vi "Stop All Plugins.vi"(8 "error in (no error)":errorcluster, 11 "CIFPluginLoader in":refnum<class "CIFPluginLoader.lvclass">) -> (0 "error out":errorcluster, 3 "CIFPluginLoader out":refnum<class "CIFPluginLoader.lvclass">)   [LabVIEW 2021, in "CIFPluginLoader.lvclass"]
uses:
  CIFPluginLoader.lvclass
  CIFPluginLoader.lvclass/CIFPluginLoader.ctl
  CIFUtilities/CIFLogs/Typedef/Message Type.ctl
  typedef/Loaded Plugin Map.ctl
  <vilib>/gRPC/LabVIEW gRPC Library/Client API/Close Client.vi
  CIFCore/Grpc/CIFCoreWrapper/CIFCoreWrapper.lvlib
  CIFUtilities/CIFLogs/CIFLogs.lvlib
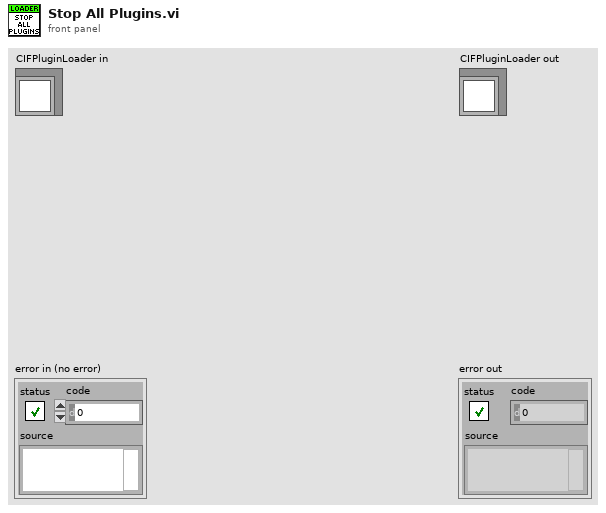
[diagram p1: front panel]
types:
  T1 = typedef "CIFPluginLoader.lvclass/Loaded Plugin Map.ctl" = map{string, refnum<vi>}
  T2 = typedef "grpc-lvsupport-release.lvlib/grpcId.ctl" = u64
  T3 = typedef "CIFLogs.lvlib/Message Type.ctl" = enum16{"Error", "Information", "Print Terminal", "Configuration"}
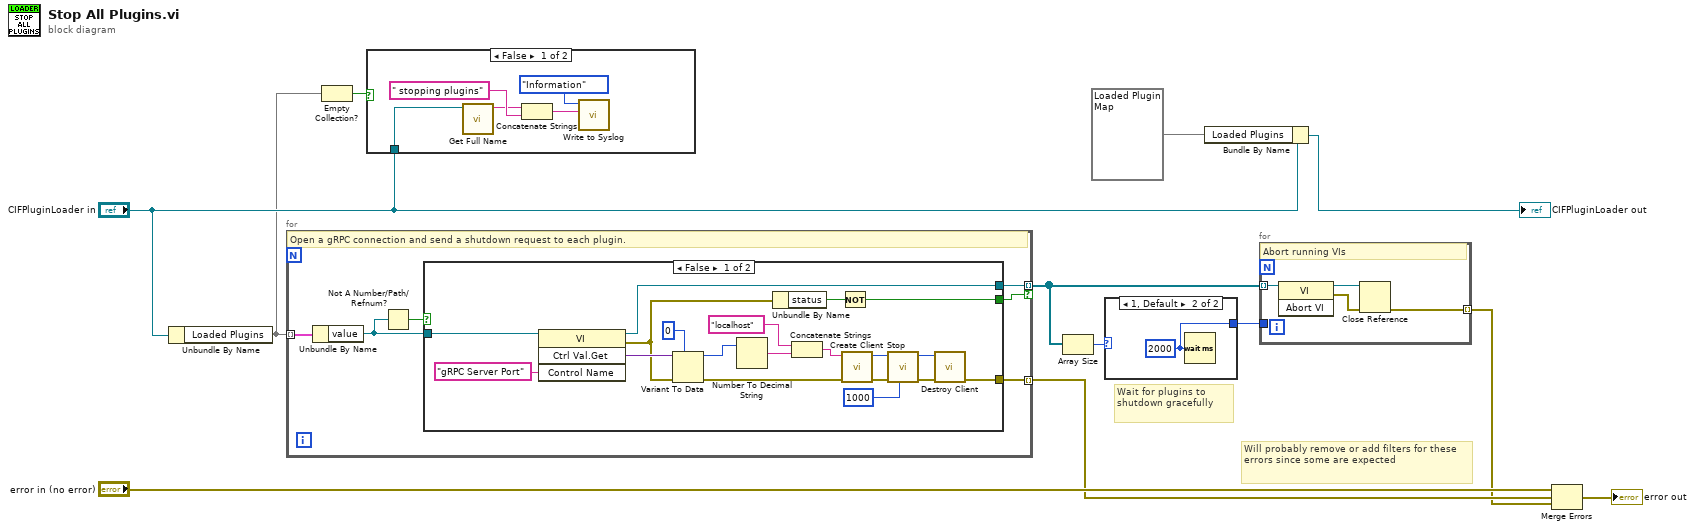
[diagram p0: block diagram]
diagram:
  # "Wait for plugins to shutdown gracefully"
  # "Will probably remove or add filters for these errors since some are expected"
  n1 = Unbundle By Name("CIFPluginLoader in") -> ("Loaded Plugins"=w1:T1)
  n2 = for {
    tunnel: w1 -> [w17] mode=indexing
    tunnel: [w15] -> w12 mode=indexing if=w14
    tunnel: [w13] -> w8 mode=indexing
    # "Open a gRPC connection and send a shutdown request to each plugin."
    n3 = Unbundle By Name(w17) -> ("value"=w16:refnum<vi>)
    n4 = Not A Number/Path/Refnum?(number/path/refnum=w16) -> (NaN/Path/Refnum?=w18:bool)
    n5 = case shown="False" w18 {
      tunnel: w16 -> [w36 _]
      tunnel: [w23 _] -> w15
      tunnel: [w20 _] -> w14
      tunnel: [w19 _] -> w13
      frame False {
        n6 = invoke class="VI" method="Ctrl Val.Get"(reference=w36, "Control Name"="gRPC Server Port") -> (reference out=w23:refnum<vi>, error out=w22:errorcluster, "Get Control Value Variant"=w35:variant)  [unwired: 2 in, 1 out]
        n7 = Variant To Data(error in=w22, type=0, Variant=w35) -> (data=w33:i32, error out=w32:errorcluster)
        n8 = Number To Decimal String(number=w33) -> (decimal integer string=w31:string)  [unwired: 1 in]
        n9 = Unbundle By Name(w22) -> ("status"=w21:bool)
        n10 = Concatenate Strings("localhost" ("string"), w31) -> (w29:string)
        n11 = Not(x=w21) -> (.not. x?=w20:bool)
        n12 = call "Create Client.vi"("error in"=w32, "address"=w29) -> ("error out"=w28:errorcluster, "gRPC ID Out"=w27:T2)  [unwired: 8 in]
        n13 = call "Stop.vi"("timeout (ms)"=1000, "error in"=w28, "gRPC ID"=w27) -> ("error out"=w24:errorcluster, "gRPC ID out"=w25:T2)  [unwired: 7 in]
        n14 = call "Destroy Client.vi"("error in"=w24, "gRPC ID"=w25) -> ("error out"=w19:errorcluster)  [unwired: 9 in]
      }
      frame True {
      }
    }
  }
  n15 = Empty Collection?(1:w1) -> (0:w2:bool)
  n16 = case shown="False" w2 {
    tunnel: "CIFPluginLoader in" -> [w38 _]
    frame False {
      n17 = call "Get Full Name.vi"("CIFPluginLoader in"=w38) -> ("Name"=w39:string)  [unwired: 10 in]
      n18 = Concatenate Strings(w39, " stopping plugins" ("message")) -> (w40:string)
      n19 = call "Write to Syslog.vi"("message"=w40, "CIF Message Type"=Message_Type."Information") -> ()  [unwired: 9 in, 1 out]
    }
    frame True {
    }
  }
  n20 = Array Size(array=w12) -> (size(s)=w11:i32)
  n21 = case shown="1, Default" w11 {
    tunnel: [_ w43] -> w10
    frame 0 {
    }
    frame 1, Default {
      w43 = u32 2000 ("milliseconds to wait")
      n22 = Wait (ms)(milliseconds to wait=w43) -> ()  [unwired: 1 out]
    }
  }
  n23 = Bundle By Name(cluster="CIFPluginLoader in", "Loaded Plugins"=T1 {}) -> (→"CIFPluginLoader out":refnum<class "CIFPluginLoader.lvclass">)
  n24 = for {
    tunnel: w12 -> [w47] mode=indexing
    tunnel: w10 -> [_]
    tunnel: [w44] -> w6 mode=indexing
    # "Abort running VIs"
    n25 = invoke class="VI" method="Abort VI"(reference=w47) -> (reference out=w46:refnum<vi>, error out=w45:errorcluster)  [unwired: 2 in, 1 out]
    n26 = Close Reference(reference=w46, error in (no error)=w45) -> (error out=w44:errorcluster)
  }
  n27 = Merge Errors("error in (no error)", w8, w6) -> (→"error out":errorcluster)
